vi "Send Write Request.vi"(8 "error in (no error)":errorcluster, 9 "Write Request":refnum<class "WriteRequest.lvclass">, 10 "Connection Manager Queue":refnum<class "Message Enqueuer.lvclass">, 11 "PersistantConnectionHandler in":refnum<class "PersistantConnectionHandler.lvclass">) -> (0 "error out":errorcluster, 3 "PersistantConnectionHandler out":refnum<class "PersistantConnectionHandler.lvclass">)   [LabVIEW 2019, in "PersitantConnectionHandler.lvlib" / "PersistantConnectionHandler.lvclass"]
uses:
  <vilib>/gpm_packages/@cs/Network-interface/Source/PersistantConnectionHandler/PersistantConnectionHandler/PersistantConnectionHandler.lvclass
  C:/Program Files/National Instruments/LabVIEW 2019/vi.lib/gpm_packages/@cs/Network-interface/Source/Logged Actor/LoggedActor.lvclass
  <vilib>/ActorFramework/Message Enqueuer/Message Enqueuer.lvclass
  <vilib>/gpm_packages/@cs/Network-interface/Source/MessagingInterfaces/WriteRequest/WriteRequest.lvclass
  <vilib>/gpm_packages/@cs/Network-interface/Source/ConnectionManager/ConnectionManager Messages/Process Write Request Msg/Process Write Request Msg.lvclass/Process Write Request Msg.ctl
  <vilib>/ActorFramework/Message Enqueuer/Message Enqueuer.lvclass/Message Enqueuer.ctl
  <vilib>/gpm_packages/@cs/event-logger/Source/Composed Log/Types/Log Level.ctl
  <vilib>/gpm_packages/@cs/Network-interface/Source/Logged Actor/LoggedActor.lvclass/LoggedActor.ctl
  <vilib>/gpm_packages/@cs/event-logger/Source/Composed Log/LoggerReference/LoggerReference.lvclass/LoggerReference.ctl
  <vilib>/ActorFramework/Message Enqueuer/Enqueue.vi
  <vilib>/gpm_packages/@cs/event-logger/Source/Composed Log/LoggerReference/Log Event.vi
  <vilib>/gpm_packages/@cs/event-logger/Source/Composed Log/LoggerReference/Log.vi
  <vilib>/gpm_packages/@cs/event-logger/Source/Composed Log/LoggerReference/Get Valid Event Time.vi
  <vilib>/gpm_packages/@cs/event-logger/Source/Composed Log/LoggerReference/Remove Stale Logs.vi
  <vilib>/gpm_packages/@cs/Network-interface/Source/ConnectionManager/ConnectionManager Messages/Process Write Request Msg/Process Write Request Msg.lvclass
  C:/Program Files/National Instruments/LabVIEW 2019/vi.lib/ActorFramework/Message/Message.lvclass
  <vilib>/ActorFramework/Message Priority Queue/Priority Enqueue.vi
  <vilib>/ErrorRing/Error Ring.xnode
  <vilib>/gpm_packages/@cs/event-logger/Source/Composed Log/Composed Log.lvlib
  <vilib>/gpm_packages/@cs/Network-interface/Source/Logged Actor/LoggedActor.lvclass
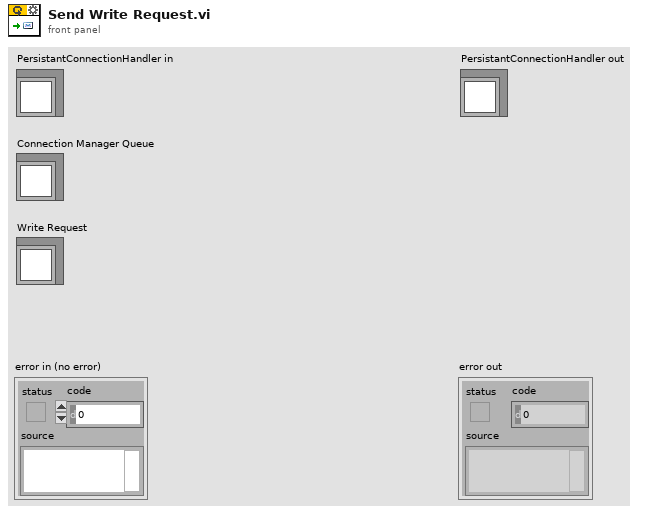
[diagram p1: front panel]
types:
  T1 = typedef "Composed Log.lvlib/Log Level.ctl" = enum16{"Debug", "Info", "Warning", "Error", "Critical"}
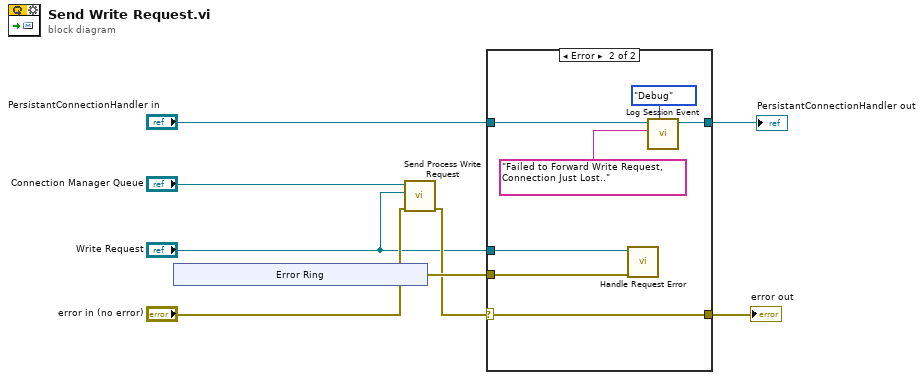
[diagram p0: block diagram]
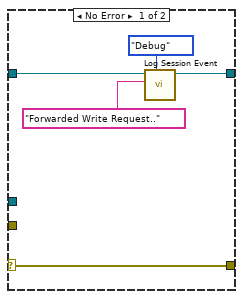
[diagram p2: hidden frame]
diagram:
  n1 = xnode "Error Ring"() -> ("error out"=w8:errorcluster)
  n2 = call <vilib>:"Send Process Write Request.vi"("error in (no error)"="error in (no error)", "Write Request"="Write Request", "Message Enqueuer"="Connection Manager Queue") -> ("error out"=w4:errorcluster)  [unwired: 7 in, 1 out]
  n3 = case shown="Error" w4 {
    selector: w4 -> [w13 w20]
    tunnel: "PersistantConnectionHandler in" -> [w12 w15]
    tunnel: [w11 w14] -> w7
    tunnel: "Write Request" -> [_ w19]
    tunnel: [w13 w20] -> w1
    tunnel: w8 -> [_ w18]
    frame No Error {
      n4 = call <vilib>:"Log Session Event.vi"("Event Level"=Log_Level."Debug", "Event Data"="Forwarded Write Request..", "SessionActor in"=w12) -> ("SessionActor out"=w11:refnum<class "PersistantConnectionHandler.lvclass">)  [unwired: 7 in, 1 out]
    }
    frame Error {
      n5 = call-dynamic "Handle Request Error.vi"("Request Error"=w18, "WriteRequest in"=w19) -> ()  [unwired: 10 in]
      n6 = call <vilib>:"Log Session Event.vi"("Event Level"=Log_Level."Debug", "Event Data"="Failed to Forward Write Request, Connection Just Lost..", "SessionActor in"=w15) -> ("SessionActor out"=w14:refnum<class "PersistantConnectionHandler.lvclass">)  [unwired: 7 in, 1 out]
    }
  }
  "error out" <- w1
  "PersistantConnectionHandler out" <- w7
